vi "표지판 없는 동적장애물.vi"(1 "2차원배열":T1) -> (0 "불리언":bool)   [LabVIEW 2016]
uses:
  <vilib>/imath/engines/lvmath2/RunTimeEngine/Managers/WorkSpace/UID Generator.vi
  <vilib>/imath/engines/lvmath2/RunTimeEngine/BuiltInFunctions/size/NIMS_I32Row=size(GM).vi
  <instcachedir>/0/NIMS_I32Row=size(GM)_10ACDCB9F1F84A7E9F42C91D87611FB5.lvgen/NIMS_I32Row=size(GM)_10ACDCB9F1F84A7E9F42C91D87611FB5_001.vi
  <vilib>/imath/engines/lvmath2/RunTimeEngine/RunTimeType/NIMS_RunTimeType_From StrictType (excl LVString).vi
  <instcachedir>/0/NIMS_RunTimeType_From StrictType (excl LVString)_BBF44FB49F834B71AF7A14CCEDF8BECD.lvgen/NIMS_RunTimeType_From StrictType (excl LVString)_BBF44FB49F834B71AF7A14CCEDF8BECD_000.vi
  <vilib>/imath/engines/lvmath2/RunTimeEngine/LocalVariableDefStatement/MC_LocalVariableDefStatement_Display.vi
  <vilib>/imath/engines/lvmath2/RunTimeEngine/IndexRead/NIMS V(S).vi
  <instcachedir>/0/NIMS V(S)_0488751826AF41519A22953C041130DC.lvgen/NIMS V(S)_0488751826AF41519A22953C041130DC_002.vi
  <vilib>/imathl/engines/lvmath/Functions/Error Handling/Create Error.vi
  <vilib>/imath/engines/lvmath2/RunTimeEngine/Managers/SymbolTable/Clear UID.vi
  <vilib>/imath/engines/lvmath2/RunTimeEngine/NodeEndStatement/NIMS_NodeEndStatement_Output.vi
  <instcachedir>/0/NIMS_NodeEndStatement_Output_53EC0D466D134D7ABD903AC30B43404B.lvgen/NIMS_NodeEndStatement_Output_53EC0D466D134D7ABD903AC30B43404B_011.vi
  <vilib>/imath/engines/lvmath2/RunTimeEngine/ErrorHandling/NIMS_Finalize Error.vi
  <vilib>/imath/engines/lvmath2/RunTimeEngine/IndexRead/NIMS M($,S).vi
  <instcachedir>/0/NIMS M($,S)_3E5749BBB62E49528D4765A77F1F6D98.lvgen/NIMS M($,S)_3E5749BBB62E49528D4765A77F1F6D98_000.vi
  <vilib>/imath/engines/lvmath2/RunTimeEngine/BuiltInFunctions/min/1 input/NIMS_min(RV).vi
  <instcachedir>/0/NIMS_min(RV)_EE2DD3E2888846108C5160A664B67832.lvgen/NIMS_min(RV)_EE2DD3E2888846108C5160A664B67832_000.vi
  <instcachedir>/0/NIMS_NodeEndStatement_Output_53EC0D466D134D7ABD903AC30B43404B.lvgen/NIMS_NodeEndStatement_Output_53EC0D466D134D7ABD903AC30B43404B_001.vi
  <vilib>/imath/engines/lvmath2/RunTimeEngine/Managers/SymbolTable/NIMS_WorkSpace.lvlib
panel:
  out "에러 출력 2":errorcluster caption="에러 출력"
  out "에러 출력":errorcluster
  out "x >= y?":bool
  out "x < y?":bool
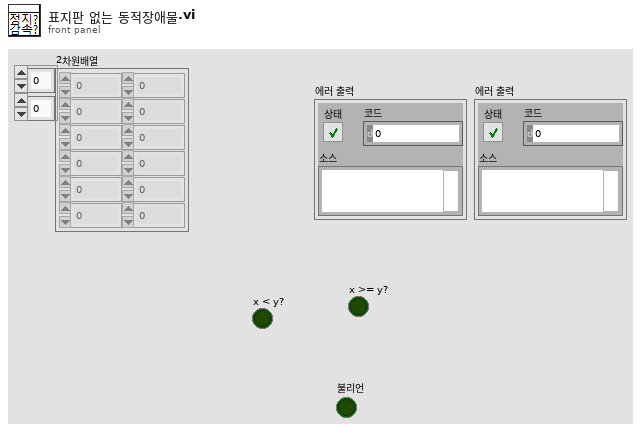
[diagram p1: front panel]
types:
  T1 = typedef "2차원배열 공유변수.ctl" = dbl[][]
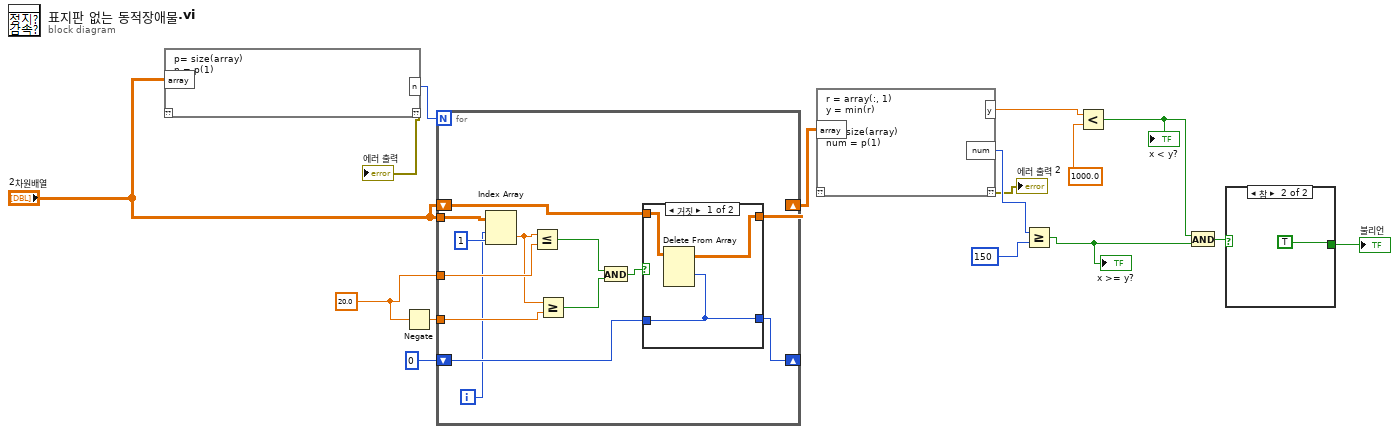
[diagram p0: block diagram]
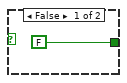
[diagram p2: hidden frame]
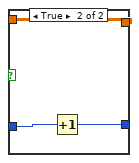
[diagram p3: hidden frame]
diagram:
  w12 = 20.0
  n1 = mathscript code="p= size(array)\nn = p(1)"("array"="2차원배열") -> ("??"=→"에러 출력":errorcluster, "n"=w15:i32)  [unwired: 1 in]
  n2 = Negate(x=w12) -> (-x=w13:dbl)
  n3 = for {
    N: w15 -> [_]
    tunnel: w12 -> [w28]
    tunnel: w13 -> [w26]
    shift-right: [w19] -> _
    shift-left: 0 ("비활성화된 인덱스 (행)") -> [w21]
    shift-right: [w20] -> w10
    shift-left: "2차원배열" -> [w22]
    tunnel: "2차원배열" -> [w18]
    i -> [w17]
    n4 = Index Array(array=w18, index (row)=w17, index (col)=1 ("비활성화된 인덱스 (열)")) -> (element=w27:dbl)
    n5 = Less Or Equal?(x=w27, y=w28) -> (x <= y?=w25:bool)
    n6 = Greater Or Equal?(x=w27, y=w26) -> (x >= y?=w24:bool)
    n7 = And(x=w25, y=w24) -> (x .and. y?=w23:bool)
    n8 = case shown="거짓" w23 {
      tunnel: w22 -> [w32 w33]
      tunnel: w21 -> [w30 w35]
      tunnel: [w31 w33] -> w20
      tunnel: [w30 w34] -> w19
      frame False {
        n9 = Delete From Array(array=w32, index (row)=w30) -> (array with subset deleted=w31:T1)  [unwired: 2 in, 1 out]
      }
      frame True {
        n10 = Increment(x=w35) -> (x+1=w34:i32)
      }
    }
  }
  n11 = mathscript code="r = array(:, 1)\ny = min(r)\n\np = size(array)\nnum = p(1)"("array"=w10) -> ("??"=→"에러 출력 2":errorcluster, "y"=w9:dbl, "num"=w4:i32)  [unwired: 1 in]
  n12 = Greater Or Equal?(x=w4, y=150) -> (x >= y?=w6:bool)
  "x >= y?" <- w6
  n13 = Less?(x=w9, y=1000.0) -> (x < y?=w7:bool)
  "x < y?" <- w7
  n14 = And(x=w7, y=w6) -> (x .and. y?=w5:bool)
  n15 = case shown="참" w5 {
    tunnel: [FALSE ("불리언") TRUE ("불리언")] -> w11
    frame False {
    }
    frame True {
    }
  }
  "불리언" <- w11
